vi "Event Read.vi"(4 "error in (no error)":errorcluster, 6 "Container State":T4, 7 "Display State In":T1={"param"=[{"min"=-100.0, "max"=150.0, "real pos"=100.0}, {"min"=-900.0, "max"=100.0, "real pos"=-100.0}, {"min"=-13.0, "max"=150.0, "real pos"=13.0}], "positions"=[0.0, 0.0, 0.0], "CellsI"=enum."5", "CellsIII"=enum."7", "step,ps"=100.0, " preset pos"=[], "event"=refnum}) -> (0 "error out":errorcluster, 2 "Value":refnum<user-event>, 3 "Display State Out":T1={"param"=[{"min"=-100.0, "max"=150.0, "real pos"=100.0}, {"min"=-900.0, "max"=100.0, "real pos"=-100.0}, {"min"=-13.0, "max"=150.0, "real pos"=13.0}], "positions"=[0.0, 0.0, 0.0], "CellsI"=enum."5", "CellsIII"=enum."7", "step,ps"=100.0, " preset pos"=[], "event"=refnum})   [LabVIEW 2020, in "ControlDL.xctl"]
uses:
  ControlDL.xctl
  <vilib>/_xctls/Container State.ctl
  stateDL.ctl
  controls/CellsSDI.ctl
  controls/CellBoolean.ctl
  controls/CellsSDIII.ctl
  <vilib>/_xctls/XControlSupport.lvlib
panel:
  # "Replace the Value Indicator below with an Indicator of desired type.\nDo not remove this Indicator or the others from the connector pane. \nDo not change the connector pane pattern.\nThe Value Indicator should always be the second terminal from top on the output side in the connector pane."
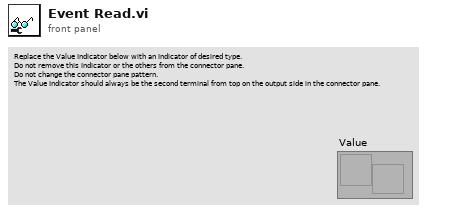
[diagram p1: front panel]
types:
  T1 = typedef "ControlDL.xctl/stateDL.ctl" = cluster{"param":cluster{"min":dbl, "max":dbl, "real pos":dbl}[], "positions":dbl[], "CellsI":T2, "CellsIII":T3, "step,ps":dbl, " preset pos":dbl[][], "event":refnum<user-event>}
  T2 = typedef "CellsSDI.ctl" = enum32{"5", "4", "3", "2", "1", "L"}
  T3 = typedef "CellsSDIII.ctl" = enum32{"7", "6", "5", "4", "3", "2", "1", "L"}
  T4 = typedef "XControlSupport.lvlib/Container State.ctl" = cluster{"Indicator?":bool, "Run Mode?":bool, " Refnum":refnum<vi>}
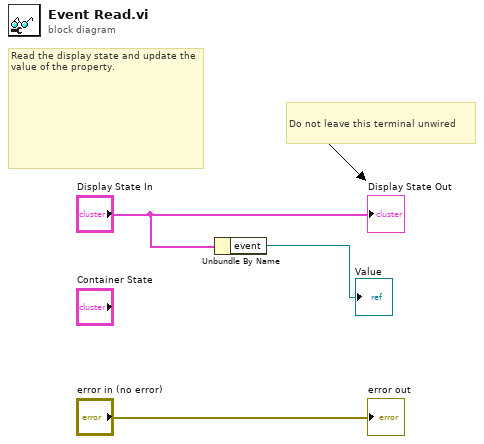
[diagram p0: block diagram]
diagram:
  # "Do not leave this terminal unwired"
  # "Read the display state and update the value of the property."
  n1 = Unbundle By Name("Display State In") -> ("event"=→"Value":refnum<user-event>)
  "error out" <- "error in (no error)"
  "Display State Out" <- "Display State In"
